vi "SetGXMLCfgDyn.vi"(8 "error in (no error)":errorcluster, 10 "DynChanCfg":T1, 11 "Dynamic in":refnum<class "Dynamic.lvclass">) -> (0 "error out":errorcluster, 3 "Dynamic out":refnum<class "Dynamic.lvclass">)   [LabVIEW 2018, in "Measurement Channels.lvlib" / "Dynamic.lvclass"]
uses:
  Dynamic.lvclass
  DynamicProps_TD.ctl
  Dynamic.lvclass/Dynamic.ctl
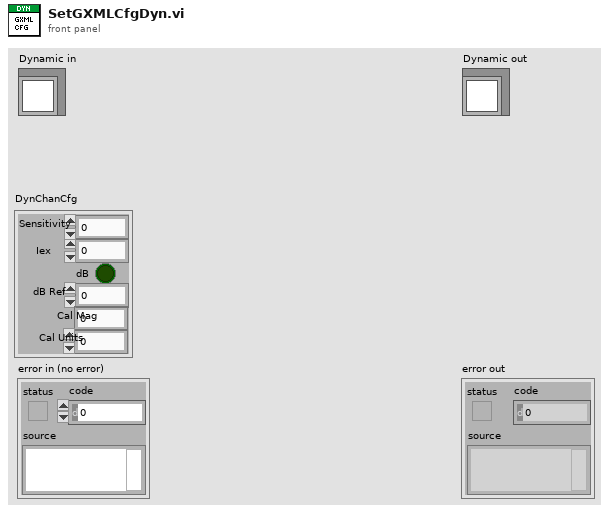
[diagram p1: front panel]
types:
  T1 = typedef "Measurement Channels.lvlib/Dynamic.lvclass/DynamicProps_TD.ctl" = cluster{"Sensitivity":dbl, "Iex":dbl, "dB":bool, "dB Ref":dbl, "Cal Mag":dbl, "Cal Units":u16}
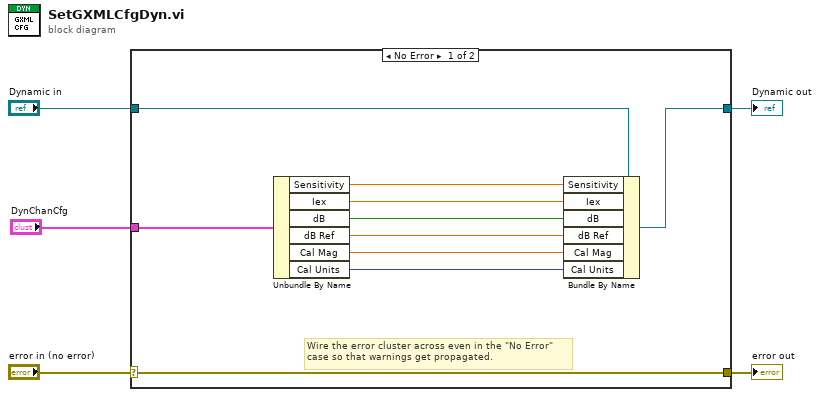
[diagram p0: block diagram]
diagram:
  n1 = case shown="No Error" "error in (no error)" {
    selector: "error in (no error)" -> [w15 w17]
    tunnel: [w15 w17] -> w4
    tunnel: [w6 w16] -> w2
    tunnel: "Dynamic in" -> [w7 w16]
    tunnel: "DynChanCfg" -> [w8 _]
    frame No Error {
      # "Wire the error cluster across even in the \"No Error\"\ncase so that warnings get propagated."
      n2 = Unbundle By Name(w8) -> ("Sensitivity"=w14:dbl, "Iex"=w13:dbl, "dB"=w12:bool, "dB Ref"=w11:dbl, "Cal Mag"=w10:dbl, "Cal Units"=w9:u16)
      n3 = Bundle By Name(cluster=w7, "Sensitivity"=w14, "Iex"=w13, "dB"=w12, "dB Ref"=w11, "Cal Mag"=w10, "Cal Units"=w9) -> (w6:refnum<class "Dynamic.lvclass">)
    }
    frame Error {
    }
  }
  "error out" <- w4
  "Dynamic out" <- w2
